vi "transform.vi"(6 "SpaceVector.lvclass":refnum<class "SpaceVector.lvclass">, 7 "zoom":dbl, 8 "error in (no error)":errorcluster, 9 "x angle (psi)":dbl[unit], 10 "z angle (phi)":dbl[unit], 11 "TrajectoryMG100122AODFrameScan in":refnum<class "TrajectoryMG100122AODFrameScan.lvclass">) -> (0 "error out":errorcluster, 3 "TrajectoryMG100122AODFrameScan out":refnum<class "TrajectoryMG100122AODFrameScan.lvclass">)   [LabVIEW 2010, in "TrajectoryMG100122AODFrameScan.lvclass"]
uses:
  TrajectoryMG100122AODFrameScan.lvclass
  common/classes/SpaceVector/SpaceVector/SpaceVector.lvclass
  TrajectoryMG100122GenericFPGA/TrajectoryMG100122GenericFPGA/TrajectoryMG100122GenericFPGA.lvclass
  FPGAWrapper/FPGAWrapperMH120124AOD/FPGAWrapperMH120124FrameScan_PXI7813R/FPGAWrapperMH120124FrameScan_PXI7813R.lvclass
  FPGAWrapper/GenericFPGAWrapper/GenericFPGAWrapper/GenericFPGAWrapper.lvclass
  TrajectoryMG100122AODFrameScan.lvclass/TrajectoryMG100122AODFrameScan.ctl
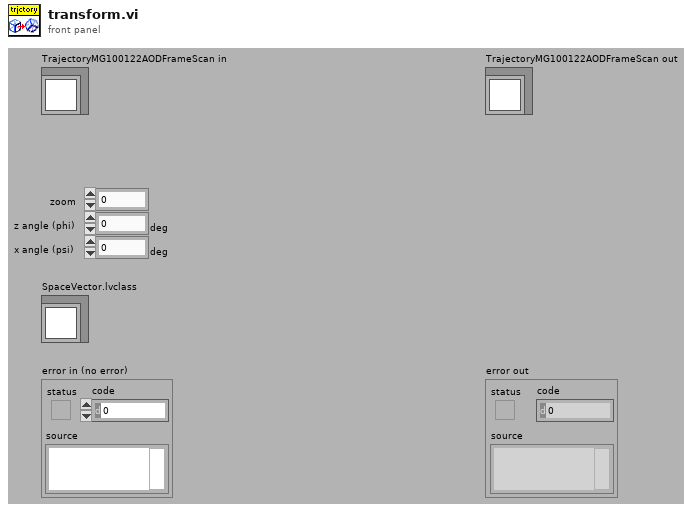
[diagram p1: front panel]
types:
  T1 = typedef "space_vector_array.ctl" = dbl[unit][]
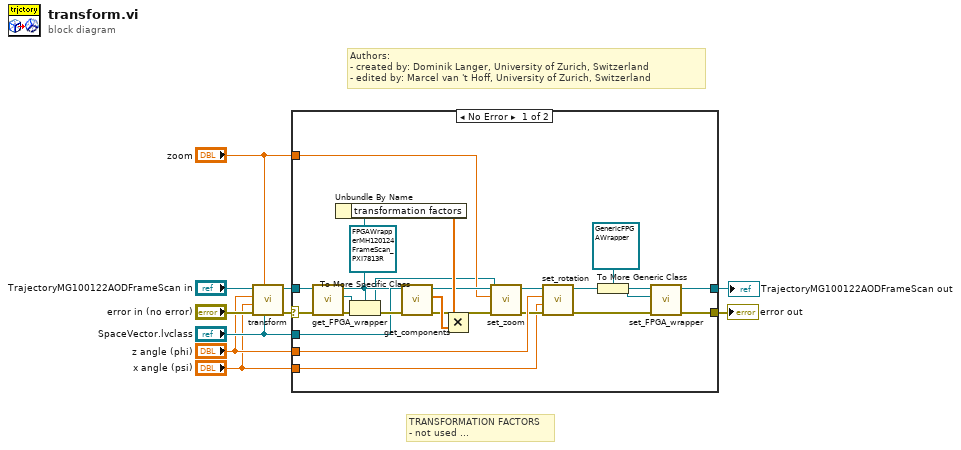
[diagram p0: block diagram]
diagram:
  # "TRANSFORMATION FACTORS\n- not used ..."
  # "Authors: \n- created by: Dominik Langer, University of Zurich, Switzerland\n- edited by: Marcel van 't Hoff, University of Zurich, Switzerland"
  n1 = call-parent "transform.vi"("SpaceVector.lvclass"="SpaceVector.lvclass", "zoom"="zoom", "error in (no error)"="error in (no error)", "x angle (psi)"="x angle (psi)", "z angle (phi)"="z angle (phi)", "TrajectoryMG100122GenericFPGA in"="TrajectoryMG100122AODFrameScan in") -> ("error out"=w8:errorcluster, "TrajectoryMG100122GenericFPGA out"=w7:refnum<class "TrajectoryMG100122AODFrameScan.lvclass">)  [unwired: 4 in]
  n2 = case shown="No Error" w8 {
    selector: w8 -> [w30 w34]
    tunnel: w7 -> [w31 w35]
    tunnel: "SpaceVector.lvclass" -> [w26 _]
    tunnel: "z angle (phi)" -> [w17 _]
    tunnel: "x angle (psi)" -> [w13 _]
    tunnel: "zoom" -> [w19 _]
    tunnel: [w25 w34] -> w2
    tunnel: [w23 w35] -> w1
    frame No Error {
      n3 = call-dynamic "get_FPGA_wrapper.vi"("error in (no error)"=w30, "TrajectoryMG100122GenericFPGA in"=w31) -> ("error out"=w28:errorcluster, "GenericFPGAWrapper.lvclass"=w29:refnum<class "GenericFPGAWrapper.lvclass">, "TrajectoryMG100122GenericFPGA out"=w24:refnum<class "TrajectoryMG100122AODFrameScan.lvclass">)  [unwired: 7 in]
      n4 = Unbundle By Name(w24) -> ("transformation factors"=w33:dbl[unit][])
      n5 = To More Specific Class(target class=refnum<class "FPGAWrapperMH120124FrameScan_PXI7813R.lvclass"> refnum ("FPGAWrapperMH120124FrameScan_PXI7813R.lvclass"), reference=w29, error in=w28) -> (specific class reference=w11:refnum<class "FPGAWrapperMH120124FrameScan_PXI7813R.lvclass">, error out=w27:errorcluster)
      n6 = call "get_components.vi"("error in (no error)"=w27, "SpaceVector in"=w26) -> ("error out"=w12:errorcluster, "x/y/z"=w32:T1)  [unwired: 4 in, 4 out]
      n7 = Multiply(x=w33, y=w32) -> ()  [unwired: 1 out]
      n8 = call-dynamic "set_zoom.vi"("error in (no error)"=w12, "zoom"=w19, "FPGAWrapperMH120124FrameScan_PXI7813R in"=w11) -> ("error out"=w16:errorcluster, "FPGAWrapperMH120124FrameScan_PXI7813R out"=w18:refnum<class "FPGAWrapperMH120124FrameScan_PXI7813R.lvclass">)  [unwired: 7 in]
      n9 = call-dynamic "set_rotation.vi"("error in (no error)"=w16, "x angle (rotation angle, phi)"=w13, "z angle (rotation angle, phi)"=w17, "FPGAWrapperMH120124FrameScan_PXI7813R in"=w18) -> ("error out"=w15:errorcluster, "FPGAWrapperMH120124FrameScan_PXI7813R out"=w14:refnum<class "FPGAWrapperMH120124FrameScan_PXI7813R.lvclass">)  [unwired: 6 in]
      n10 = To More Generic Class(target class=refnum<class "GenericFPGAWrapper.lvclass"> refnum ("GenericFPGAWrapper.lvclass"), reference=w14) -> (generic class reference=w22:refnum<class "GenericFPGAWrapper.lvclass">)
      n11 = call-dynamic "set_FPGA_wrapper.vi"("error in (no error)"=w15, "GenericFPGAWrapper.lvclass"=w22, "TrajectoryMG100122GenericFPGA in"=w24) -> ("error out"=w25:errorcluster, "TrajectoryMG100122GenericFPGA out"=w23:refnum<class "TrajectoryMG100122AODFrameScan.lvclass">)  [unwired: 7 in]
    }
    frame Error {
    }
  }
  "error out" <- w2
  "TrajectoryMG100122AODFrameScan out" <- w1
